vi "Get LabVIEW Error Message.vi"(1 "Error Cluster":errorcluster) -> (0 "Error Message":string)   [LabVIEW 2016]
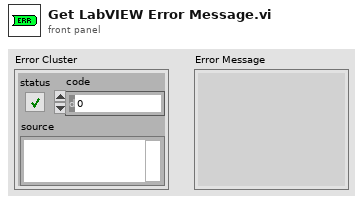
[diagram p1: front panel]
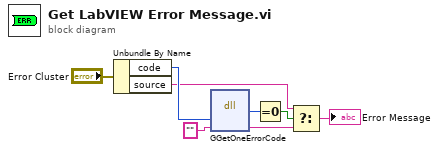
[diagram p0: block diagram]
diagram:
  n1 = Unbundle By Name("Error Cluster") -> ("code"=w4:i32, "source"=w3:string)
  n2 = dll-call lib="LabVIEW" fn="GGetOneErrorCode"("errorCode"=w4, "" ("input param")) -> (w7:u8, w5:string)  [unwired: 4 in, 2 out]
  n3 = Equal To 0?(x=w7) -> (x = 0?=w6:bool)
  n4 = Select(t=w3, s=w6, f=w5) -> (s? t:f=→"Error Message":string)
